vi "Launcher Engine Type Specifier.vi"(0 "Unique Notifier Name":string, 11 "Device Ports/IDs/Channels":string[](array[string])) -> ()   [LabVIEW 2016]
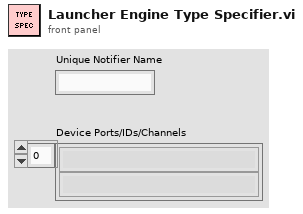
[diagram p1: front panel]
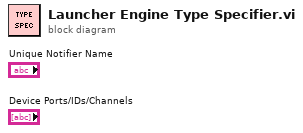
[diagram p0: block diagram]
diagram:
